vi "Merge Map.vi"(8 "error in (no error)":errorcluster, 11 "Map Model in":refnum<class "Map Model.lvclass">) -> (0 "error out":errorcluster, 2 "Map":picture, 3 "Map Model out":refnum<class "Map Model.lvclass">)   [LabVIEW 2020, in "Map Model.lvlib" / "Map Model.lvclass"]
uses:
  Map Model.lvclass
  Map Model.lvclass/Map Model.ctl
panel:
  # "NOTICE -- YOU MUST LEAVE THIS NOTICE IN PLACE.\n\nCopyright (c) 2017, LIANG LIU Shawn.Liu.cn@gmail.com\nAll rights reserved.\n\nRedistribution and use in source and binary forms, with or without modification, are permitted provided that the following conditions are met:\n-Redistributions of source code must retain the above copyright notice, this list of conditions and the following disclaimer.\n-Redistributions in binary form must reproduce the above copyright notice, this list of conditions and the following disclaimer in the documentation and/or other materials provided with the distribution.\n-Neither the name of the eLp nor the names of its contributors may be used to endorse or promote products derived from this software without specific prior written permission.\n\nTHIS SOFTWARE IS PROVIDED BY THE COPYRIGHT HOLDERS AND CONTRIBUTORS \"AS IS\" AND ANY EXPRESS OR IMPLIED WARRANTIES, INCLUDING, BUT NOT LIMITED TO, THE IMPLIED WARRANTIES OF MERCHANTABILITY AND FITNESS FOR A PARTICULAR PURPOSE ARE DISCLAIMED. IN NO EVENT SHALL THE COPYRIGHT HOLDER OR CONTRIBUTORS BE LIABLE FOR ANY DIRECT, INDIRECT, INCIDENTAL, SPECIAL, EXEMPLARY, OR CONSEQUENTIAL DAMAGES (INCLUDING, BUT NOT LIMITED TO, PROCUREMENT OF SUBSTITUTE GOODS OR SERVICES; LOSS OF USE, DATA, OR PROFITS; OR BUSINESS INTERRUPTION) HOWEVER CAUSED AND ON ANY THEORY OF LIABILITY, WHETHER IN CONTRACT, STRICT LIABILITY, OR TORT (INCLUDING NEGLIGENCE OR OTHERWISE) ARISING IN ANY WAY OUT OF THE USE OF THIS SOFTWARE, EVEN IF ADVISED OF THE POSSIBILITY OF SUCH DAMAGE."
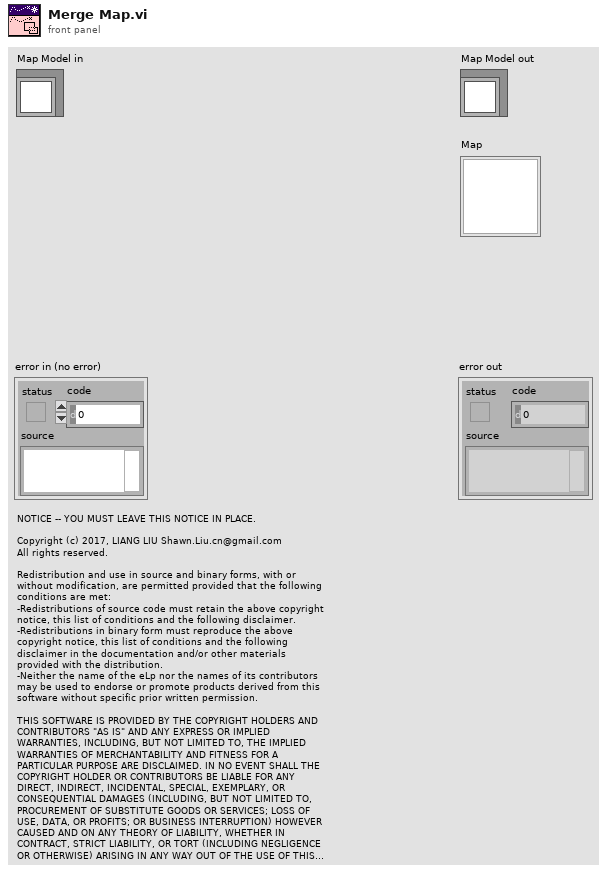
[diagram p1: front panel]
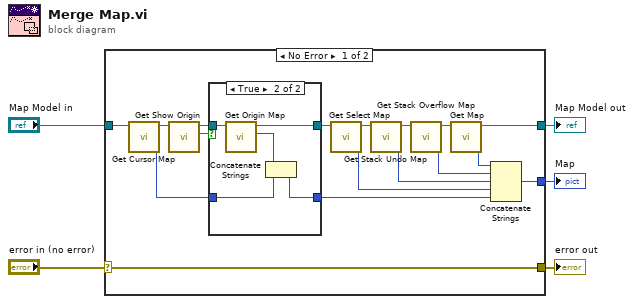
[diagram p0: block diagram]
diagram:
  n1 = case shown="No Error" "error in (no error)" {
    selector: "error in (no error)" -> [w19 w31]
    tunnel: [w22 _] -> w5
    tunnel: "Map Model in" -> [w21 w30]
    tunnel: [w20 w30] -> w3
    tunnel: [w19 w31] -> w1
    frame No Error {
      n2 = call "Get Cursor Map.vi"("Map Model in"=w21) -> ("Cursor Map"=w7:picture, "Map Model out"=w15:refnum<class "Map Model.lvclass">)  [unwired: 9 in]
      n3 = call "Get Show Origin.vi"("Map Model in"=w15) -> ("Show Origin"=w9:bool, "Map Model out"=w13:refnum<class "Map Model.lvclass">)  [unwired: 9 in]
      n4 = case shown="True" w9 {
        tunnel: w13 -> [w23 w29]
        tunnel: [w23 w28] -> w12
        tunnel: [w24 w25] -> w8
        tunnel: w7 -> [w24 w26]
        frame False {
        }
        frame True {
          n5 = call "Get Origin Map.vi"("Map Model in"=w29) -> ("Origin Map"=w27:picture, "Map Model out"=w28:refnum<class "Map Model.lvclass">)  [unwired: 9 in]
          n6 = Concatenate Strings(w27, w26) -> (w25:picture)
        }
      }
      n7 = call "Get Select Map.vi"("Map Model in"=w12) -> ("Select Map"=w10:picture, "Map Model out"=w11:refnum<class "Map Model.lvclass">)  [unwired: 9 in]
      n8 = call "Get Stack Undo Map.vi"("Map Model in"=w11) -> ("Stack Undo Map"=w17:picture, "Map Model out"=w16:refnum<class "Map Model.lvclass">)  [unwired: 9 in]
      n9 = call "Get Stack Overflow Map.vi"("Map Model in"=w16) -> ("Stack Overflow Map"=w18:picture, "Map Model out"=w6:refnum<class "Map Model.lvclass">)  [unwired: 9 in]
      n10 = call "Get Map.vi"("Map Model in"=w6) -> ("Map"=w14:picture, "Map Model out"=w20:refnum<class "Map Model.lvclass">)  [unwired: 9 in]
      n11 = Concatenate Strings(w14, w18, w17, w10, w8) -> (w22:picture)
    }
    frame Error {
    }
  }
  "error out" <- w1
  "Map Model out" <- w3
  "Map" <- w5
